vi "XSP3_GetAllData_v2.vi"(6 "NumRoi":i32=1, 8 "ErrorIn":errorcluster, 9 "NumCh":i32=1, 11 "ProcessIn":string="XSPRESS3-EXAMPLE" caption="ProcessName") -> (0 "ErrorOut":errorcluster, 2 "Status":bool, 3 "ProcessOut":string caption="ProcessName", 4 "Data":T1)   [LabVIEW 2010]
uses:
  Program Files/National Instruments/LabVIEW 2017/user.lib/caLab/Private/Get_PV-1D.vi
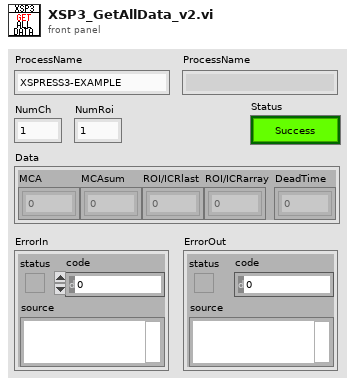
[diagram p1: front panel]
types:
  T1 = cluster{"MCA":dbl[][], "MCAsum":dbl[][], "ROI/ICRlast":dbl[], "ROI/ICRarray":dbl[][], "DeadTime":dbl[]}
  T2 = cluster{"Value Array (number)":dbl[][], "Value Array (number)":dbl[][], "Value Array (number)":dbl[], "Value Array (number)":dbl[][], "Value Array (number)":dbl[]}
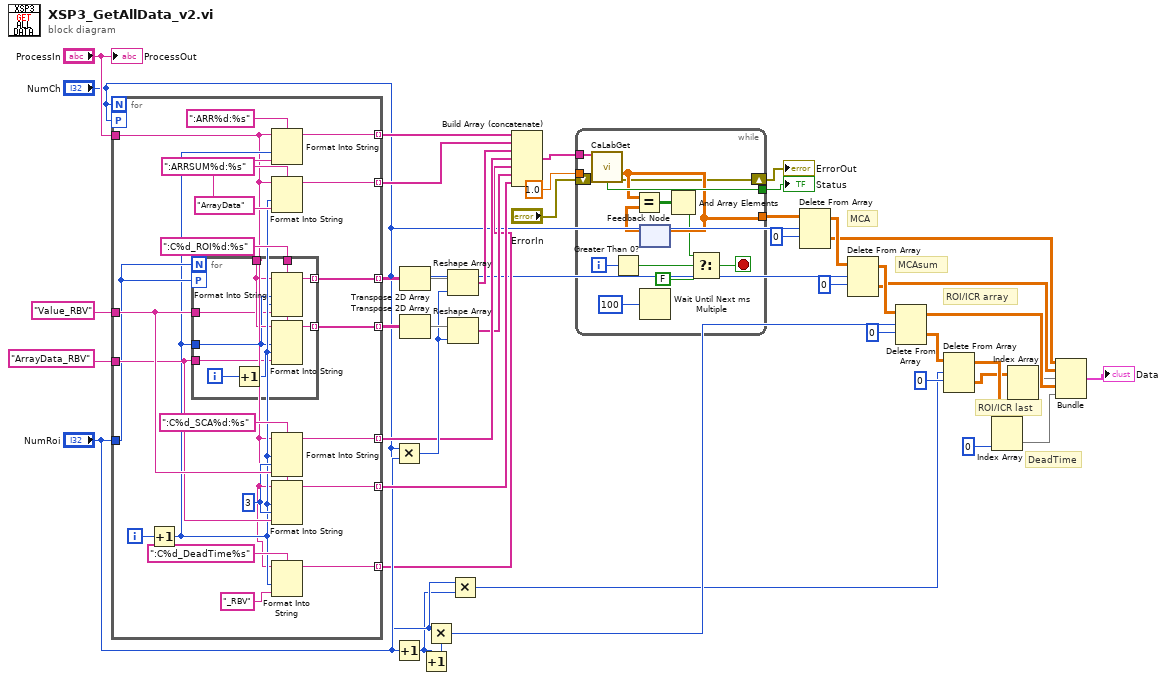
[diagram p0: block diagram]
diagram:
  # "DeadTime"
  # "ROI/ICR array"
  # "ROI/ICR last"
  # "MCAsum"
  # "MCA"
  n1 = for {
    N: "NumCh" -> [_]
    tunnel: "ProcessIn" -> [w44]
    tunnel: "NumRoi" -> [w57]
    tunnel: "Value_RBV" ("PV") -> [w63]
    tunnel: "ArrayData_RBV" ("PV") -> [w62]
    workers-P: "NumCh" -> [_]
    tunnel: [w56] -> w36 mode=indexing
    tunnel: [w55] -> w35 mode=indexing
    tunnel: [w54] -> w21 mode=indexing
    tunnel: [w53] -> w19 mode=indexing
    tunnel: [w52] -> w34 mode=indexing
    tunnel: [w51] -> w33 mode=indexing
    tunnel: [w45] -> w6 mode=indexing
    i -> [w64]
    w49 = 3 ("input 2")
    w59 = "ArrayData" ("PV")
    w61 = ":C%d_SCA%d:%s" ("PV")
    n2 = Increment(x=w64) -> (x+1=w46:i32)
    n3 = for {
      N: w57 -> [_]
      tunnel: w44 -> [w73]
      tunnel: w46 -> [w70]
      tunnel: w63 -> [w69]
      tunnel: w62 -> [w68]
      tunnel: [w67] -> w52 mode=indexing
      tunnel: [w66] -> w51 mode=indexing
      workers-P: w57 -> [_]
      tunnel: ":C%d_ROI%d:%s" ("PV") -> [w65]
      i -> [w72]
      n4 = Increment(x=w72) -> (x+1=w71:i32)
      n5 = Format Into String(format string=w65, initial string=w73, w70, w71, w69) -> (resulting string=w67:string)  [unwired: 1 in, 1 out]
      n6 = Format Into String(format string=w65, initial string=w73, w70, w71, w68) -> (resulting string=w66:string)  [unwired: 1 in, 1 out]
    }
    n7 = Format Into String(format string=":ARR%d:%s" ("PV"), initial string=w44, w46, w59) -> (resulting string=w56:string)  [unwired: 1 in, 1 out]
    n8 = Format Into String(format string=":ARRSUM%d:%s" ("PV"), initial string=w44, w46, w59) -> (resulting string=w55:string)  [unwired: 1 in, 1 out]
    n9 = Format Into String(format string=w61, initial string=w44, w46, w49, w63) -> (resulting string=w54:string)  [unwired: 1 in, 1 out]
    n10 = Format Into String(format string=w61, initial string=w44, w46, w49, w62) -> (resulting string=w53:string)  [unwired: 1 in, 1 out]
    n11 = Format Into String(format string=":C%d_DeadTime%s" ("PV"), initial string=w44, w46, "_RBV" ("PV")) -> (resulting string=w45:string)  [unwired: 1 in, 1 out]
  }
  n12 = Multiply(x="NumCh", y="NumRoi") -> (x*y=w24:i32)
  n13 = Increment(x="NumRoi") -> (x+1=w4:i32)
  n14 = Transpose 2D Array(2D array=w34) -> (transposed array=w26:string[][])
  n15 = Transpose 2D Array(2D array=w33) -> (transposed array=w25:string[][])
  n16 = Increment(x=w4) -> (x+1=w9:i32)
  n17 = Multiply(x="NumCh", y=w9) -> (x*y=w8:i32)
  n18 = Reshape Array(w26, w24) -> (w22:string[])
  n19 = Reshape Array(w25, w24) -> (w20:string[])
  n20 = Multiply(x="NumCh", y=w4) -> (x*y=w3:i32)
  n21 = Build Array (concatenate)(w36, w35, w22, w21, w6, w20, w19) -> (w32:string[])
  n22 = while {
    tunnel: 1.0 ("Timeout (3)") -> [w87]
    tunnel: [w86] -> w40
    tunnel: w32 -> [w85]
    shift-right: [w74] -> w41
    shift-left: "ErrorIn" -> [w75]
    tunnel: [w82] -> w14
    i -> [w76]
    stop <- w80 stop-if-true
    n23 = call-poly "CaLabGet.vi"("PV Names"=w85, "Timeout (3)"=w87, "Error in (no error)"=w75) -> ("Value Array (number)"=w82:dbl[][], "Status"=w86:bool, "Error out"=w74:errorcluster)  [unwired: 6 in, 4 out]
    n24 = Greater Than 0?(x=w76) -> (x > 0?=w77:bool)
    n25 = feedback-in #1(w82) -> ()
    n26 = feedback #1() -> (w83:dbl[][])  [unwired: 1 in]
    n27 = Equal?(x=w82, y=w83) -> (x = y?=w84:bool[][])
    n28 = Wait Until Next ms Multiple(millisecond multiple=u32 100) -> ()  [unwired: 1 out]
    n29 = And Array Elements(Boolean array=w84) -> (logical AND=w78:bool)
    n30 = Select(t=w78, s=w77, f=FALSE) -> (s? t:f=w80:bool)
  }
  "ErrorOut" <- w41
  "Status" <- w40
  n31 = Delete From Array(array=w14, length="NumCh", index (row)=0) -> (deleted portion=w18:dbl[][], array with subset deleted=w29:dbl[][])  [unwired: 1 in]
  n32 = Delete From Array(array=w29, length="NumCh", index (row)=0) -> (deleted portion=w17:dbl[][], array with subset deleted=w27:dbl[][])  [unwired: 1 in]
  n33 = Delete From Array(array=w27, length=w8, index (row)=0) -> (deleted portion=w13:dbl[][], array with subset deleted=w16:dbl[][])  [unwired: 1 in]
  n34 = Delete From Array(array=w13, length=w3, index (row)=0) -> (deleted portion=w1:dbl[][], array with subset deleted=w2:dbl[][])  [unwired: 1 in]
  n35 = Index Array(array=w2, index (col)=0 ("disabled index (col)")) -> (element=w11:dbl[])  [unwired: 1 in]
  n36 = Index Array(array=w1) -> (element=w10:dbl[])  [unwired: 2 in]
  n37 = Bundle("Value Array (number)"=w18, "Value Array (number)"=w17, "Value Array (number)"=w10, "Value Array (number)"=w16, "Value Array (number)"=w11) -> (→"Data":T2)  [unwired: 1 in]
  "ProcessOut" <- "ProcessIn"
